vi "resampleAndCombine(SubVI).vi"(3 "ATI data":waveform(dbl)[](array[waveform]), 4 "resample dt (s)":dbl, 5 "PS data":waveform(dbl)[](array[waveform])) -> (1 "all Data":dbl[][](array[numeric]))   [LabVIEW 2017]
uses:
  <vilib>/measure/maresamp.llb/Resample Waveform (single shot).vi
  <vilib>/measure/NI_MAPro.lvlib
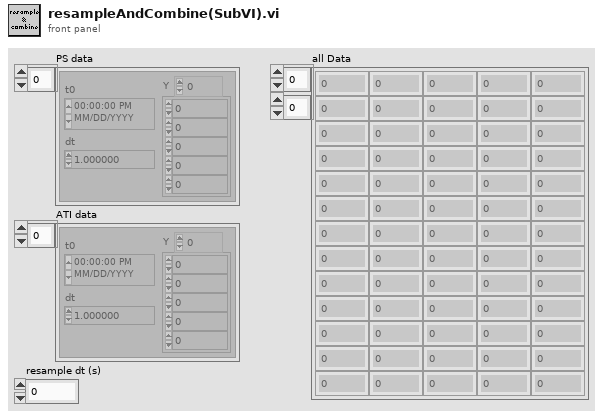
[diagram p1: front panel]
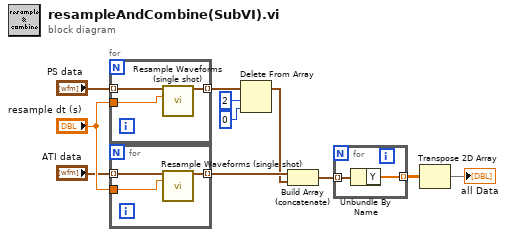
[diagram p0: block diagram]
diagram:
  n1 = for {
    tunnel: "PS data" -> [w14] mode=indexing
    tunnel: [w13] -> w5 mode=indexing
    tunnel: "resample dt (s)" -> [w12]
    n2 = call-poly <vilib>:"Resample Waveforms (single shot).vi"("waveform in"=w14, "dt"=w12) -> ("resampled waveform out"=w13:waveform(dbl))  [unwired: 10 in, 3 out]
  }
  n3 = for {
    tunnel: "ATI data" -> [w17] mode=indexing
    tunnel: [w16] -> w8 mode=indexing
    tunnel: "resample dt (s)" -> [w15]
    n4 = call-poly <vilib>:"Resample Waveforms (single shot).vi"("waveform in"=w17, "dt"=w15) -> ("resampled waveform out"=w16:waveform(dbl))  [unwired: 10 in, 3 out]
  }
  n5 = Delete From Array(array=w5, length=2, index=0) -> (array with subset deleted=w7:waveform(dbl)[])  [unwired: 1 out]
  n6 = Build Array (concatenate)(w8, w7) -> (w9:waveform(dbl)[])
  n7 = for {
    tunnel: w9 -> [w19] mode=indexing
    tunnel: [w18] -> w10 mode=indexing
    n8 = Unbundle By Name(w19) -> ("Y"=w18:dbl[])
  }
  n9 = Transpose 2D Array(2D array=w10) -> (transposed array=→"all Data":dbl[][])
